vi "create test channels.vi"() -> (0 "error out":errorcluster, 1 "names":string[](array[string]), 2 "chans":refnum<class "TBM channel.lvclass">[](array[class]), 3 "TDMS datalogger configuration out":refnum<class "TDMS datalogger configuration.lvclass">)   [LabVIEW 2013, in "tdms logger tests.lvlib"]
uses:
  tdms logger tests.lvlib
  <vilib>/NI/Tag Bus Module Framework/channel/channel classification.ctl
  <vilib>/NI/Tag Bus Module Framework/channel/TBM channel.lvclass
  configuration/TDMS datalogger configuration.lvclass
  <vilib>/NI/Configuration Framework/serializable configuration/NISE_CEF_serializable configuration.lvclass
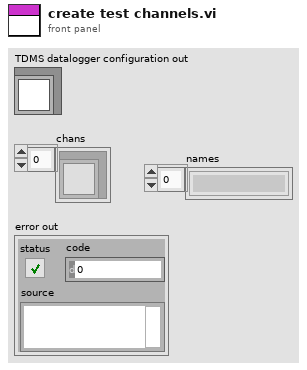
[diagram p1: front panel]
types:
  T1 = typedef "tag bus.lvlib/tag descriptor.lvclass/Data Type.ctl" = enum16{"Double", "Single", "I64", "I32", "I16", "I8", "U64", "U32", "U16", "U8", "Boolean", "String", "Array of Double", "Array of Single", "Array of I64", "Array of I32", "Array of I16", "Array of I8", "Array of U64", "Array of U32", "Array of U16", "Array of U8", "Array of Boolean", "Array of String"}
  T2 = typedef "TBM channel.lvclass/channel classification.ctl" = enum16{"input data", "output data", "processing parameter", "processing result"}
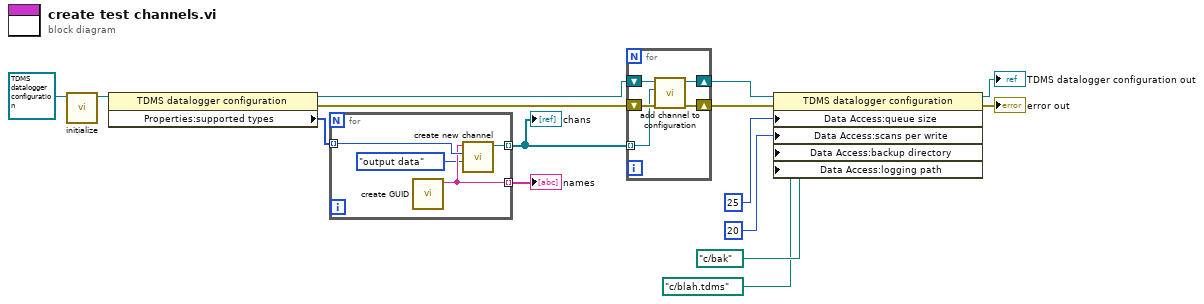
[diagram p0: block diagram]
diagram:
  n1 = call <vilib>:"initialize.vi"("configuration in"=refnum<class "TDMS datalogger configuration.lvclass"> refnum ("TDMS datalogger configuration")) -> ("configuration out"=w10:refnum<class "TDMS datalogger configuration.lvclass">)  [unwired: 8 in, 2 out]
  n2 = property class="TDMS datalogger configuration"(reference=w10) -> (reference out=w13:refnum<class "TDMS datalogger configuration.lvclass">, error out=w14:errorcluster, "Properties:supported types"=w11:T1[])  [unwired: 1 in]
  n3 = for {
    tunnel: [w19] -> w15 mode=indexing
    tunnel: w11 -> [w18] mode=indexing
    tunnel: [w17] -> w9 mode=indexing
    n4 = call <vilib>:"create GUID.vi"() -> ("uuid"=w17:string)  [unwired: 10 in, 1 out]
    n5 = call <vilib>:"create new channel.vi"("channel classification"=channel_classification."output data", "data type"=w18, "channel name"=w17) -> ("channel"=w19:refnum<class "TBM channel.lvclass">)  [unwired: 8 in]
  }
  "chans" <- w15
  "names" <- w9
  n6 = for {
    shift-right: [w23] -> w4
    shift-left: w13 -> [w24]
    shift-right: [w21] -> w1
    shift-left: w14 -> [w22]
    tunnel: w15 -> [w20] mode=indexing
    n7 = call "add channel to configuration.vi"("error in"=w22, "TBM channel in"=w20, "TDMS datalogger configuration in"=w24) -> ("error out"=w21:errorcluster, "TDMS datalogger configuration out"=w23:refnum<class "TDMS datalogger configuration.lvclass">)  [unwired: 7 in]
  }
  n8 = property class="TDMS datalogger configuration"(reference=w4, error in=w1, "Data Access:queue size"=25 ("queue size"), "Data Access:scans per write"=20 ("scans per write"), "Data Access:backup directory"=path "c:/bak" ("backup directory"), "Data Access:logging path"=path "c:/blah.tdms" ("logging path")) -> (reference out=→"TDMS datalogger configuration out":refnum<class "TDMS datalogger configuration.lvclass">, error out=→"error out":errorcluster)
